vi "progra 6.vi"() -> ()   [LabVIEW 2011]
panel:
  out "Alarma":bool
  out "Thermometer":i32(slide) scale=0.0..100.0
  out "Cuarta":bool
  out "Segunda":bool
  out "Tercera":bool
  out "Primera":bool
  out "Velocidad":i32(knob) scale=0.0..180.0
  # "Debera de generar la velocidad en numero entero.\nLuego de acuerdo a la siguiente tabla:\n1-30 primera\n31-50- segunda\n51-85 tercera\n86-180 cuarta\nDebera de encender las luces de los cambios"
  # "Encender alarma cuando la temperatura sobrepasa\nlos 80 grados y la velocidad es mayor a 150"
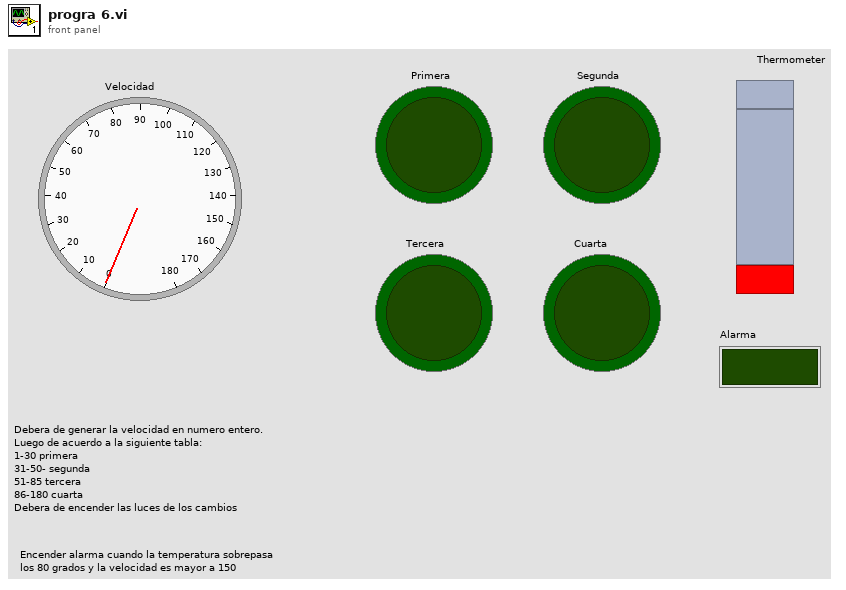
[diagram p1: front panel]
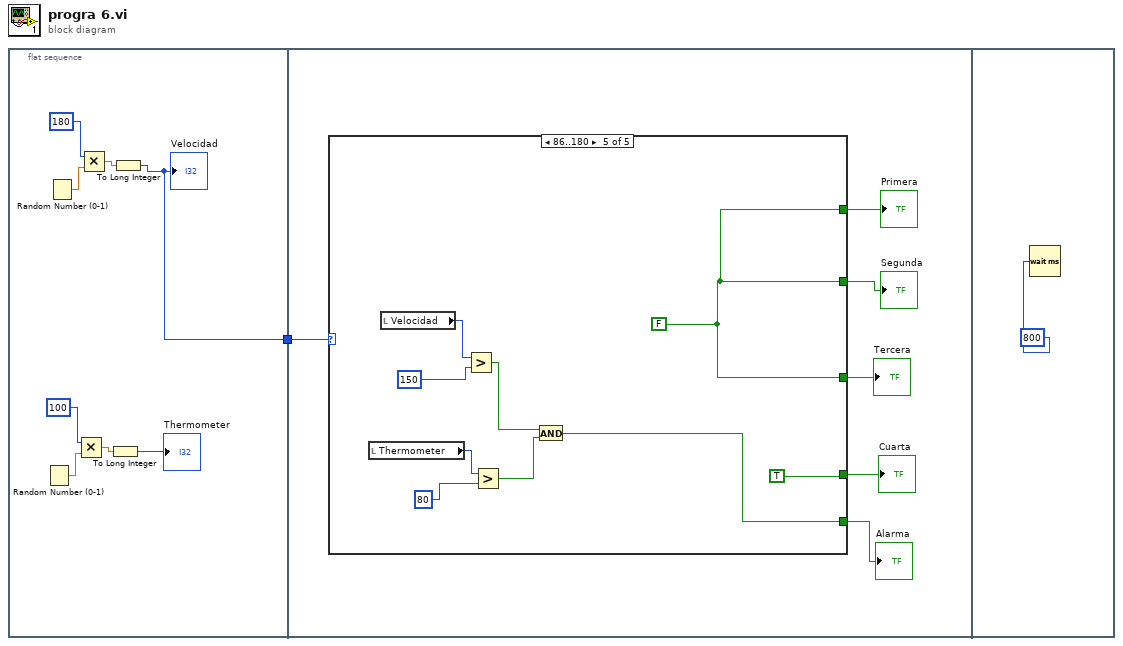
[diagram p0: block diagram]
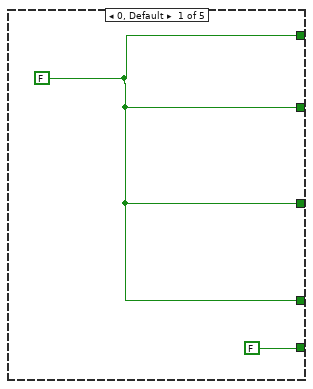
[diagram p2: hidden frame]
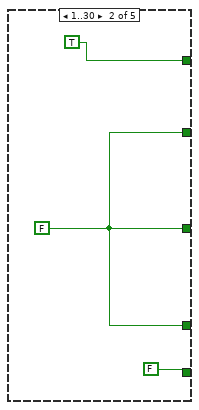
[diagram p3: hidden frame]
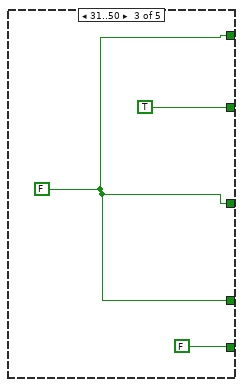
[diagram p4: hidden frame]
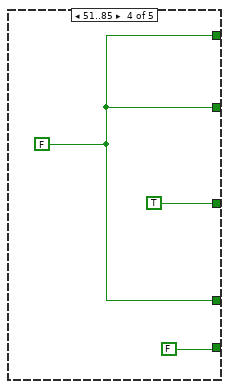
[diagram p5: hidden frame]
diagram:
  n1 = flat-sequence {
    tunnel: [w2] -> w1
    tunnel: w1 -> [w11]
    frame #0 {
      n2 = Random Number (0-1)() -> (number: 0 to 1=w9:dbl)
      n3 = Random Number (0-1)() -> (number: 0 to 1=w3:dbl)
      n4 = Multiply(x=100, y=w9) -> (x*y=w7:dbl)
      n5 = Multiply(x=180, y=w3) -> (x*y=w5:dbl)
      n6 = To Long Integer(number=w7) -> (32bit integer=→"Thermometer":i32)
      n7 = To Long Integer(number=w5) -> (32bit integer=w2:i32)
      "Velocidad" <- w2
    }
    frame #1 {
      n8 = case shown="86..180" w11 {
        tunnel: [w17 TRUE w22 w25 w34] -> w15
        tunnel: [w17 w19 TRUE w25 w34] -> w14
        tunnel: [w17 w19 w22 TRUE w34] -> w13
        tunnel: [w17 w19 w22 w25 TRUE] -> w12
        tunnel: [FALSE FALSE FALSE FALSE w27] -> w10
        frame 0, Default {
          w17 = FALSE
        }
        frame 1..30 {
          w19 = FALSE
        }
        frame 31..50 {
          w22 = FALSE
        }
        frame 51..85 {
          w25 = FALSE
        }
        frame 86..180 {
          w34 = FALSE
          n9 = local read "Thermometer"() -> (w30:i32)
          n10 = local read "Velocidad"() -> (w32:i32)
          n11 = Greater?(x=w32, y=150) -> (0:w29:bool)
          n12 = Greater?(x=w30, y=80) -> (0:w28:bool)
          n13 = And(x=w29, y=w28) -> (x .and. y?=w27:bool)
        }
      }
      "Primera" <- w15
      "Tercera" <- w13
      "Segunda" <- w14
      "Cuarta" <- w12
      "Alarma" <- w10
    }
    frame #2 {
      n14 = Wait (ms)(milliseconds to wait=800) -> ()  [unwired: 1 out]
    }
  }
